vi "CSM_Global_Init.vi"(11 "Object":T1) -> ()   [LabVIEW 2014]
uses:
  <resource>/Framework/Providers/API/ItemRef.ctl
  <resource>/Framework/Providers/API/mxLvMenuItem.ctl
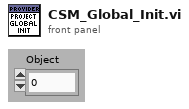
[diagram p1: front panel]
types:
  T1 = typedef "ItemRef.ctl" = u64
  T2 = typedef "mxLvMenuItem.ctl" = cluster{"Menu Name":string, "Description":string, "Icon File Name":path, "Menu Tag":string, "Enabled":bool, "Checked":bool, "Separator":bool, "Batchable":bool, "Weight":i32, "Batch Mode (Ignored if Not Batchable)":enum32{"Show If All Items Support Command", "Show If Any Items Support Command"}, "Menu Location":enum32{"<None>", "Project", "Project / Build Specifications", "Tools", "Tools / Source Control", "Tools / Real-Time Module", "Help"}, "Exclude From Getting Started Window Menu":bool}
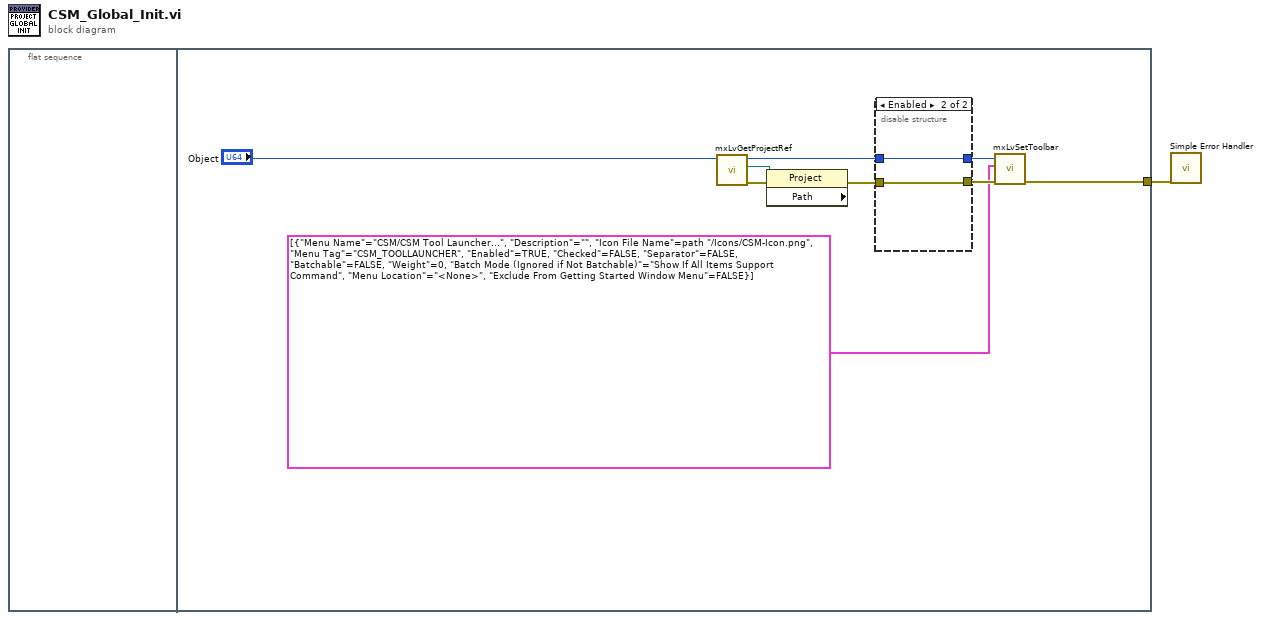
[diagram p0: block diagram]
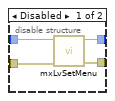
[diagram p2: hidden frame]
diagram:
  n1 = flat-sequence {
    tunnel: [w10] -> w1
    frame #0 {
    }
    frame #1 {
      n2 = call <resource>:"mxLvGetProjectRef.vi"("Item"="Object") -> ("error out"=w6:errorcluster, "Project Refnum"=w5:refnum<vi>, "Item"=w4:T1)  [unwired: 8 in]
      n3 = property class="Project" props=["Path"](reference=w5, error in=w6) -> (error out=w3:errorcluster)  [unwired: 2 out]
      n4 = disable-structure shown="Enabled" {
        disable-tunnel: [w14 w15] -> w8
        disable-tunnel: [w13 w16] -> w7
        disable-tunnel: w4 -> [w12 w15]
        disable-tunnel: w3 -> [w11 w16]
        frame Disabled {
          n5 = call <resource>:"mxLvSetMenu.vi"("error in"=w11, "Item"=w12) -> ("error out"=w13:errorcluster, "Item"=w14:T1)  [unwired: 1 in, 7 out]
        }
        frame Enabled {
        }
      }
      n6 = call <resource>:"mxLvSetToolbar.vi"("error in"=w7, "Toolbar Items"=T2[] [{"Menu Name"="CSM/CSM Tool Launcher...", "Description"="", "Icon File Name"=path "../Icons/CSM-Icon.png", "Menu Tag"="CSM_TOOLLAUNCHER", "Enabled"=TRUE, "Checked"=FALSE, "Separator"=FALSE, "Batchable"=FALSE, "Weight"=0, "Batch Mode (Ignored if Not Batchable)"=enum."Show If All Items Support Command", "Menu Location"=enum."<None>", "Exclude From Getting Started Window Menu"=FALSE}] ("Array in"), "Item"=w8) -> ("error out"=w10:errorcluster)  [unwired: 7 in, 1 out]
    }
  }
  n7 = call <vilib>:"Simple Error Handler.vi"("error in (no error)"=w1) -> ()  [unwired: 4 in, 5 out]
